vi "5.11- OCU TCP Send Client.vi"() -> ()   [LabVIEW 2010]
doc: "Displays data sent via TCP from Data Server.vi. Once a TCP connection is open, the VI reads 4 bytes to determine the amount of data being sent. It then reads and charts that many bytes. If an error occurs or the stop button is pressed, it sends a \"Q\" to the Data Sender to notify it to quit.\n\n<B>Note:</B> Requires the Data Server.vi located in the same library as this VI."
uses:
  5.0-Global.vi
panel:
  in  "Port":u16=7832 min=1025 step=1
  # "Instructions:\n1. Open the Data Server.vi located in the same library.\n2. Follow the instructions on it's front panel.\n\nNote: This VI is built to work with the Data Server.vi."
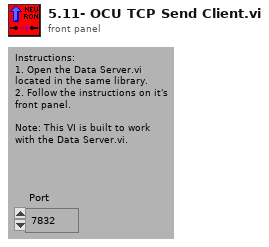
[diagram p1: front panel]
types:
  T1 = typedef "6.8-Forbrain to OCU neuron.ctl" = cluster{"6.2-Where Am I? Sensor":T2, "6.1.11-Forebrain Act Neuron Data":T5, "6.4 How Reporting":T7}
  T2 = typedef "4.2-Where Sensor Typedef.ctl" = cluster{"4.2.2- Current GPS Data":T3, "4.2.1-VectorNav Data":T4, "4.2.1-VectorNav Status":string}
  T3 = typedef "Current GPS Data.ctl" = cluster{"Lattitude (Decimal Degrees)":ext, "Longitude (Decimal Degrees)":ext, "EST Time":timestamp}
  T4 = typedef "3.2.1-VectorNav Data.ctl" = cluster{"Yaw":dbl, "Pitch":dbl, "Roll":dbl}
  T5 = typedef "6.1.11- Forbrain and midbrain Act neuron.ctl" = cluster{"4.1- Midbrain Act Data":T6, "6.1.8-Advanced VFH":dbl[]}
  T6 = typedef "4.1-Midbrain Act Data.ctl" = cluster{"Arbitrated Array":sgl[], "Exploded Obstacles":sgl[], "Desired Change in Heading":sgl, "Desired Speed Fraction":sgl}
  T7 = typedef "6.4-How Reporting Typedef.ctl" = cluster{"Drive Speed (m/s)":dbl, "Lidar Inclination (deg) ":dbl, "Steering Angle (deg)":dbl, "Battery Voltage":dbl, "Drive Encoder Cable Check":bool, "Lidar Drive Encoder Cable Check":bool, "Steer Encoder Cable Check":bool, "Lidar Pos Encoder Cable Check":bool, "Mod Buttons & Blinky Cable Check":bool, "Lidar Data Cable Check":bool, "Drive Motor Cable Check":bool, "Vector Nav Cable Check":bool, "Lidar Drive Cable Check":bool, "Steer Drive Cable Check":bool, "Reverse?":bool, "Steering Control Voltage":dbl, "Drive Control Voltage":dbl, "Lidar Control Voltage":dbl}
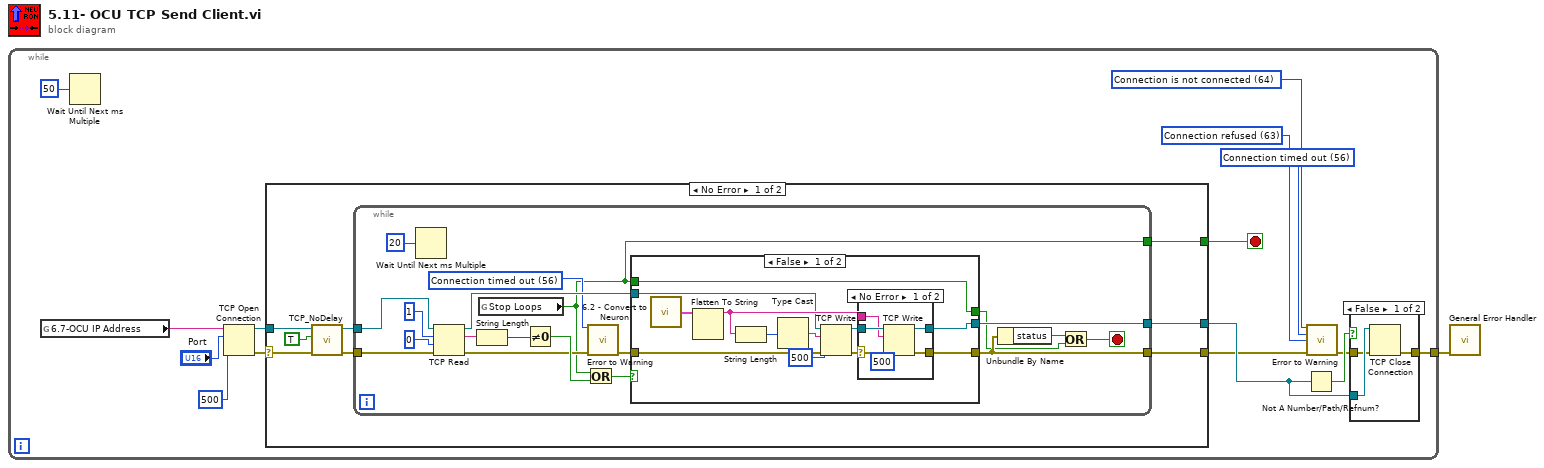
[diagram p0: block diagram]
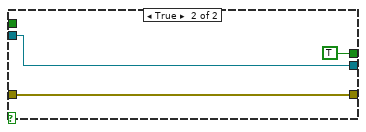
[diagram p4: hidden frame]
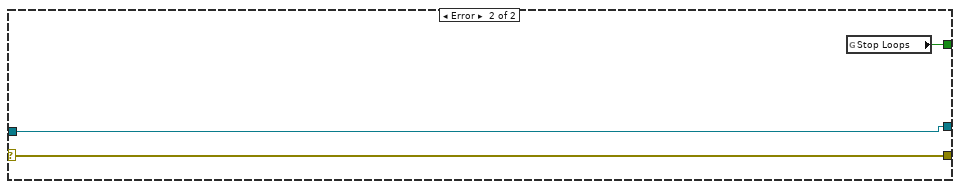
[diagram p5: hidden frame]
diagram:
  n1 = while {
    tunnel: [w6] -> w1
    stop <- w12 stop-if-true
    w3 = 56 items=["No Error", "Argument Error", "Memory Full", "Out of Zone", "End of File", "File Already Open", "Generic File IO Error", "File Not Found", "File Permission Error", "Disk Full", "Duplicate Path", "Too Many Files Open", "Not Enabled", "Resource File Not Found", "Cannot Add Resource", "Resource Not Found", "Image Not Found", "Image Memory Error", "Pen Does Not Exist", "Config Bad Type", "Config Token Not Found", "Config Parse Error", "Config Memory Error", "Bad External Code Format", "Bad External Code Offset", "External Code Not Present", "Null Window", "Destroy Window Mixup", "Null Menu", "Print Aborted", "Bad Print Record", "Print Driver Error", "Windows Error During Print", "Memory Error During Print", "Print Dialog Error", "Generic Print Error", "Invalid Device Refnum", "Device Not Found", "Device Parameter Error", "Device Unit Error", "Can't Open Device", "Device Call Aborted", "Generic Error", "Cancelled By User", "Object ID Too Low", "Object ID Too High", "Object Not In Heap", "Unknown Heap", "Bad DefProc ID", "DefProc Not In Table", "Message Out Of Range", "Null Method", "Unknown Message", "Manager Call Not Supported", "Bad address", "Connection In progress", "Connection timed out", "Connection is already in progress", "Network attribute not supported", "Network error", "Address in use", "System out of memory", "Connection aborted", "Connection refused", "Connection is not connected", "Connection is already connected", "Connection closed", "Initialize error (interapplication manager)", "Bad occurrence", "Wait on unbound occurrence handler", "Occurrence queue overflow", "Bad path", "Semaphore not signaled", "Unrecognized type (interapplication manager)"] ("2nd Error to Convert")
    w5 = 63 items=["No Error", "Argument Error", "Memory Full", "Out of Zone", "End of File", "File Already Open", "Generic File IO Error", "File Not Found", "File Permission Error", "Disk Full", "Duplicate Path", "Too Many Files Open", "Not Enabled", "Resource File Not Found", "Cannot Add Resource", "Resource Not Found", "Image Not Found", "Image Memory Error", "Pen Does Not Exist", "Config Bad Type", "Config Token Not Found", "Config Parse Error", "Config Memory Error", "Bad External Code Format", "Bad External Code Offset", "External Code Not Present", "Null Window", "Destroy Window Mixup", "Null Menu", "Print Aborted", "Bad Print Record", "Print Driver Error", "Windows Error During Print", "Memory Error During Print", "Print Dialog Error", "Generic Print Error", "Invalid Device Refnum", "Device Not Found", "Device Parameter Error", "Device Unit Error", "Can't Open Device", "Device Call Aborted", "Generic Error", "Cancelled By User", "Object ID Too Low", "Object ID Too High", "Object Not In Heap", "Unknown Heap", "Bad DefProc ID", "DefProc Not In Table", "Message Out Of Range", "Null Method", "Unknown Message", "Manager Call Not Supported", "Bad address", "Connection In progress", "Connection timed out", "Connection is already in progress", "Network attribute not supported", "Network error", "Address in use", "System out of memory", "Connection aborted", "Connection refused", "Connection is not connected", "Connection is already connected", "Connection closed", "Initialize error (interapplication manager)", "Bad occurrence", "Wait on unbound occurrence handler", "Occurrence queue overflow", "Bad path", "Semaphore not signaled", "Unrecognized type (interapplication manager)"] ("3rd Error to Convert")
    w11 = 64 items=["No Error", "Argument Error", "Memory Full", "Out of Zone", "End of File", "File Already Open", "Generic File IO Error", "File Not Found", "File Permission Error", "Disk Full", "Duplicate Path", "Too Many Files Open", "Not Enabled", "Resource File Not Found", "Cannot Add Resource", "Resource Not Found", "Image Not Found", "Image Memory Error", "Pen Does Not Exist", "Config Bad Type", "Config Token Not Found", "Config Parse Error", "Config Memory Error", "Bad External Code Format", "Bad External Code Offset", "External Code Not Present", "Null Window", "Destroy Window Mixup", "Null Menu", "Print Aborted", "Bad Print Record", "Print Driver Error", "Windows Error During Print", "Memory Error During Print", "Print Dialog Error", "Generic Print Error", "Invalid Device Refnum", "Device Not Found", "Device Parameter Error", "Device Unit Error", "Can't Open Device", "Device Call Aborted", "Generic Error", "Cancelled By User", "Object ID Too Low", "Object ID Too High", "Object Not In Heap", "Unknown Heap", "Bad DefProc ID", "DefProc Not In Table", "Message Out Of Range", "Null Method", "Unknown Message", "Manager Call Not Supported", "Bad address", "Connection In progress", "Connection timed out", "Connection is already in progress", "Network attribute not supported", "Network error", "Address in use", "System out of memory", "Connection aborted", "Connection refused", "Connection is not connected", "Connection is already connected", "Connection closed", "Initialize error (interapplication manager)", "Bad occurrence", "Wait on unbound occurrence handler", "Occurrence queue overflow", "Bad path", "Semaphore not signaled", "Unrecognized type (interapplication manager)"] ("1st Error to Convert")
    n2 = global read "5.0-Global.vi" "6.7-OCU IP Address"() -> (w4:string)
    n3 = Wait Until Next ms Multiple(millisecond multiple=u32 50) -> ()  [unwired: 1 out]
    n4 = TCP Open Connection(address=w4, remote port or service name="Port", timeout ms (60000)=500) -> (connection ID=w15:refnum<k5>, error out=w14:errorcluster)  [unwired: 1 in, 1 out]
    n5 = case shown="No Error" w14 {
      selector: w14 -> [w24 w71]
      tunnel: w15 -> [w27 w72]
      tunnel: [w28 w73] -> w12
      tunnel: [w22 w72] -> w8
      tunnel: [w21 w71] -> w7
      frame No Error {
        n6 = call "TCP_NoDelay.vi"("error in (no error)"=w24, "TCP_NODELAY (true)"=TRUE, "connID"=w27) -> ("error out"=w25:errorcluster, "connID 2"=w26:refnum<k5>)  [unwired: 3 in]
        n7 = while {
          tunnel: [w30] -> w28
          tunnel: [w39] -> w21
          tunnel: w26 -> [w32]
          tunnel: [w34] -> w22
          tunnel: w25 -> [w33]
          stop <- w47 stop-if-true
          w37 = 56 items=["No Error", "Argument Error", "Memory Full", "Out of Zone", "End of File", "File Already Open", "Generic File IO Error", "File Not Found", "File Permission Error", "Disk Full", "Duplicate Path", "Too Many Files Open", "Not Enabled", "Resource File Not Found", "Cannot Add Resource", "Resource Not Found", "Image Not Found", "Image Memory Error", "Pen Does Not Exist", "Config Bad Type", "Config Token Not Found", "Config Parse Error", "Config Memory Error", "Bad External Code Format", "Bad External Code Offset", "External Code Not Present", "Null Window", "Destroy Window Mixup", "Null Menu", "Print Aborted", "Bad Print Record", "Print Driver Error", "Windows Error During Print", "Memory Error During Print", "Print Dialog Error", "Generic Print Error", "Invalid Device Refnum", "Device Not Found", "Device Parameter Error", "Device Unit Error", "Can't Open Device", "Device Call Aborted", "Generic Error", "Cancelled By User", "Object ID Too Low", "Object ID Too High", "Object Not In Heap", "Unknown Heap", "Bad DefProc ID", "DefProc Not In Table", "Message Out Of Range", "Null Method", "Unknown Message", "Manager Call Not Supported", "Bad address", "Connection In progress", "Connection timed out", "Connection is already in progress", "Network attribute not supported", "Network error", "Address in use", "System out of memory", "Connection aborted", "Connection refused", "Connection is not connected", "Connection is already connected", "Connection closed", "Initialize error (interapplication manager)", "Bad occurrence", "Wait on unbound occurrence handler", "Occurrence queue overflow", "Bad path", "Semaphore not signaled", "Unrecognized type (interapplication manager)"] ("1st Error to Convert")
          n8 = Wait Until Next ms Multiple(millisecond multiple=u32 20) -> ()  [unwired: 1 out]
          n9 = TCP Read(connection ID=w32, bytes to read=1, error in (no error)=w33, 9:0) -> (connection ID out=w43:refnum<k5>, data out=w44:string, error out=w36:errorcluster)  [unwired: 1 in]
          n10 = String Length(string=w44) -> (length=w42:i32)
          n11 = global read "5.0-Global.vi" "Stop Loops"() -> (w30:bool)
          n12 = Not Equal To 0?(x=w42) -> (x != 0?=w41:bool)
          n13 = Or(x=w30, y=w41) -> (x .or. y?=w40:bool)
          n14 = call <vilib>:"Error to Warning.vi"("1st Error to Convert"=w37, "error in"=w36) -> ("warning out"=w35:errorcluster)  [unwired: 13 in]
          n15 = case shown="False" w40 {
            tunnel: w35 -> [w56 w68]
            tunnel: w43 -> [w52 w69]
            tunnel: [w55 w69] -> w34
            tunnel: [w54 w68] -> w39
            tunnel: [w50 TRUE] -> w29
            tunnel: w30 -> [w50 _]
            frame False {
              n16 = call "6.2 - Convert to Neuron.vi"() -> ("6.7-Forebrain to OCU Neuron"=w49:T1)
              n17 = Flatten To String(anything=w49) -> (data string=w53:string)  [unwired: 3 in, 2 out]
              n18 = String Length(string=w53) -> (length=w58:i32)
              n19 = Type Cast(x=w58) -> (*(type *) &x=w59:string)  [unwired: 1 in]
              n20 = TCP Write(connection ID=w52, data in=w59, error in (no error)=w56, 9:500 ("timeout ms (25000)")) -> (connection ID out=w57:refnum<k5>, error out=w51:errorcluster)  [unwired: 1 out]
              n21 = case shown="No Error" w51 {
                selector: w51 -> [w63 w66]
                tunnel: w57 -> [w65 w67]
                tunnel: [w61 w67] -> w55
                tunnel: [w62 w66] -> w54
                tunnel: w53 -> [w64 _]
                frame No Error {
                  n22 = TCP Write(connection ID=w65, data in=w64, error in (no error)=w63, 9:500 ("timeout ms (25000)")) -> (connection ID out=w61:refnum<k5>, error out=w62:errorcluster)  [unwired: 1 out]
                }
                frame Error {
                }
              }
            }
            frame True {
            }
          }
          n23 = Unbundle By Name(w39) -> ("status"=w38:bool)
          n24 = Or(x=w38, y=w29) -> (x .or. y?=w47:bool)
        }
      }
      frame Error {
        n25 = global read "5.0-Global.vi" "Stop Loops"() -> (w73:bool)
      }
    }
    n26 = Not A Number/Path/Refnum?(number/path/refnum=w8) -> (NaN/Path/Refnum?=w10:bool)
    n27 = call <vilib>:"Error to Warning.vi"("1st Error to Convert"=w11, "2nd Error to Convert"=w3, "3rd Error to Convert"=w5, "error in"=w7) -> ("warning out"=w9:errorcluster)  [unwired: 11 in]
    n28 = case shown="False" w10 {
      tunnel: w8 -> [w19 _]
      tunnel: w9 -> [w18 w20]
      tunnel: [w17 w20] -> w6
      frame False {
        n29 = TCP Close Connection(connection ID=w19, error in (no error)=w18) -> (error out=w17:errorcluster)  [unwired: 2 out]
      }
      frame True {
      }
    }
  }
  n30 = call <vilib>:"General Error Handler.vi"("error in (no error)"=w1) -> ()  [unwired: 2 in, 13 out]
